vi "Create.vi"(8 "error in (no error)":errorcluster, 10 "Configuration":T1={"Modes of operation"=8, "Feed(pulse)"=1000000, "Max motor speed(r/min)"=200, "Max torque(0.1%)"=500, "Min position limit(pulse)"=-2147483648, "Max position limit(pulse)"=2147483647} {"Modes of operation" items=["No mode change/no mode assigned"=0, "Profile position mode"=1, "Velocity mode"=2, "Profile velocity mode"=3, "Torque profile mode"=4, "Homing mode"=6, "Interpolated position mode"=7, "Cyclic synchronous position mode"=8, "Cyclic synchronous velocity mode"=9, "Cyclic synchronous torque mode"=10]}, 11 "Connect Info":T2) -> (0 "error out":errorcluster, 3 "Motor Base out":refnum<class "Motor Base.lvclass">)   [LabVIEW 2016, in "Motor Base.lvlib" / "Motor Base.lvclass"]
doc: "如果Configuration不会填，请参见电机手册查看数据名词解释。"
uses:
  Motor Base.lvclass
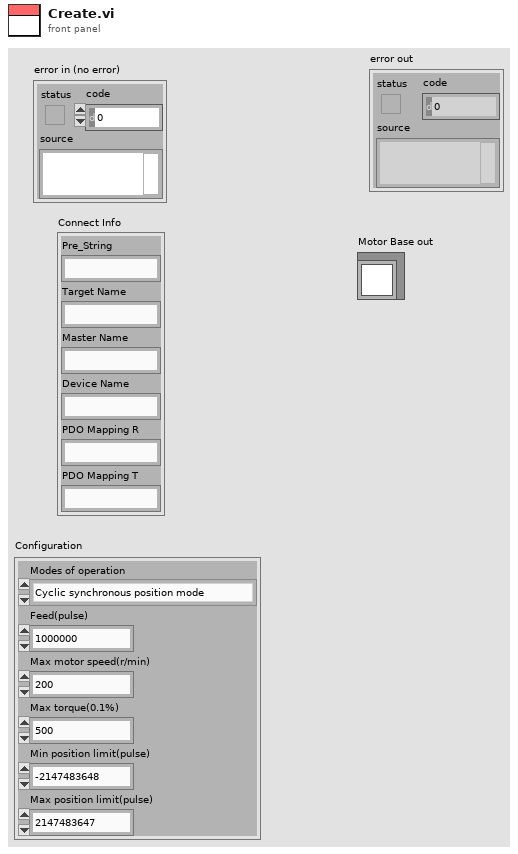
[diagram p1: front panel]
types:
  T1 = cluster{"Modes of operation":i8, "Feed(pulse)":u32, "Max motor speed(r/min)":u32, "Max torque(0.1%)":u16, "Min position limit(pulse)":i32, "Max position limit(pulse)":i32}
  T2 = cluster{"Pre_String":string, "Target Name":string, "Master Name":string, "Device Name":string, "PDO Mapping R":string, "PDO Mapping T":string}
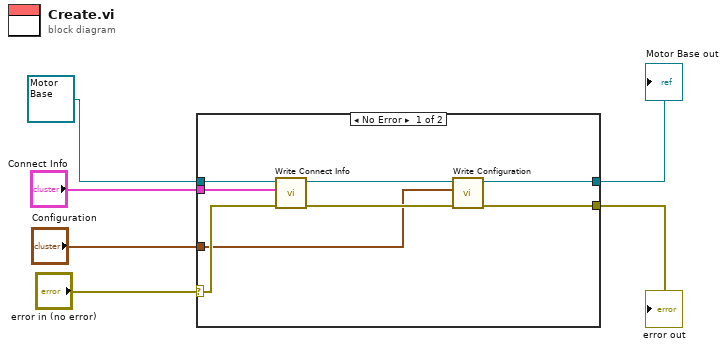
[diagram p0: block diagram]
diagram:
  n1 = case shown="No Error" "error in (no error)" {
    selector: "error in (no error)" -> [w12 w16]
    tunnel: refnum<class "Motor Base.lvclass"> refnum ("Motor Base in") -> [w14 w15]
    tunnel: "Connect Info" -> [w13 _]
    tunnel: [w10 w15] -> w4
    tunnel: [w8 w16] -> w3
    tunnel: "Configuration" -> [w7 _]
    frame No Error {
      n2 = call-dynamic "Write Connect Info.vi"("error in (no error)"=w12, "Connect Info"=w13, "Motor Base in"=w14) -> ("error out"=w9:errorcluster, "Motor Base out"=w11:refnum<class "Motor Base.lvclass">)  [unwired: 7 in]
      n3 = call-dynamic "Write Configuration.vi"("error in (no error)"=w9, "Configuration"=w7, "Motor Base in"=w11) -> ("error out"=w8:errorcluster, "Motor Base out"=w10:refnum<class "Motor Base.lvclass">)  [unwired: 7 in]
    }
    frame Error {
    }
  }
  "Motor Base out" <- w4
  "error out" <- w3
